vi "Create (From Structure).vi"(8 "error in (no error)":errorcluster, 10 "Structure":refnum<vi>) -> (0 "error out":errorcluster, 3 "JKI SM out":refnum<class "JKI SM.lvclass">)   [LabVIEW 2013, in "JKI State Machine API.lvlib" / "JKI SM.lvclass"]
uses:
  JKI SM.lvclass
  JKI SM.lvclass/JKI SM.ctl
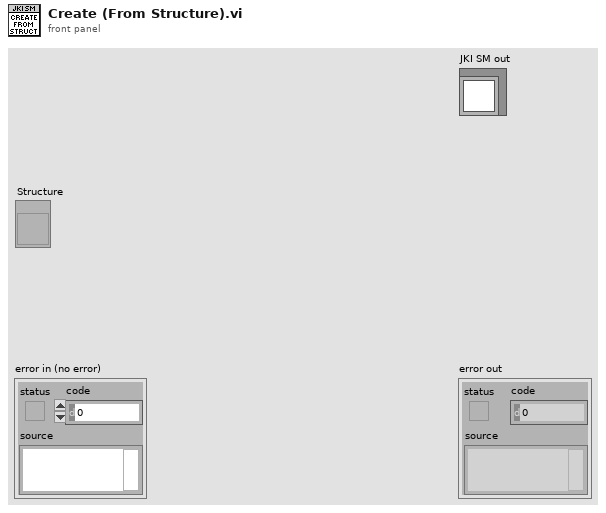
[diagram p1: front panel]
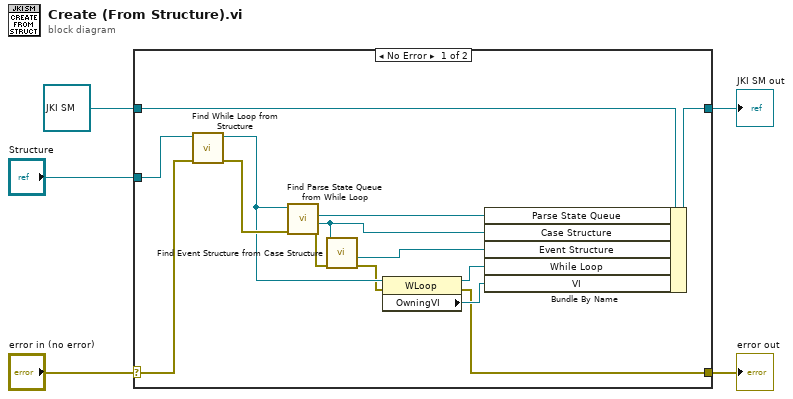
[diagram p0: block diagram]
diagram:
  n1 = case shown="No Error" "error in (no error)" {
    selector: "error in (no error)" -> [w12 w21]
    tunnel: [w6 w21] -> w4
    tunnel: [w18 w20] -> w2
    tunnel: refnum<class "JKI SM.lvclass"> refnum ("JKI SM") -> [w19 w20]
    tunnel: "Structure" -> [w13 _]
    frame No Error {
      n2 = call "Find While Loop from Structure.vi"("error in (no error)"=w12, "MultiFrameStructure in"=w13) -> ("error out"=w11:errorcluster, "WLoop Refnum"=w9:refnum<vi>)  [unwired: 8 in]
      n3 = call "Find Parse State Queue from While Loop.vi"("error in (no error)"=w11, "WhileLoop in"=w9) -> ("error out"=w14:errorcluster, "CaseStructure"=w16:refnum<vi>, "Parse State Queue"=w17:refnum<vi>)  [unwired: 7 in]
      n4 = call "Find Event Structure from Case Structure.vi"("error in (no error)"=w14, "CaseStructure"=w16) -> ("error out"=w7:errorcluster, "EvntStruct Refnum"=w15:refnum<vi>)  [unwired: 8 in]
      n5 = property class="WLoop"(reference=w9, error in=w7) -> (reference out=w8:refnum<vi>, error out=w6:errorcluster, "OwningVI"=w10:refnum<vi>)
      n6 = Bundle By Name(cluster=w19, "Parse State Queue"=w17, "Case Structure"=w16, "Event Structure"=w15, "While Loop"=w8, "VI"=w10) -> (w18:refnum<class "JKI SM.lvclass">)
    }
    frame Error {
    }
  }
  "error out" <- w4
  "JKI SM out" <- w2
